vi "Save Settings.vi"(6 "Enable":bool, 8 "error in":errorcluster, 10 "Cluster":T1, 11 "VISA Refnum in":refnum<visa-resource-name>) -> (0 "error out":errorcluster, 2 "Cluster Out":T1, 3 "VISA out":refnum<visa-resource-name>)   [LabVIEW 2020]
uses:
  f6da1217-3e19-4b15-bc5f-b1b6cffed974.vi
  WriteSingleCoil.vi
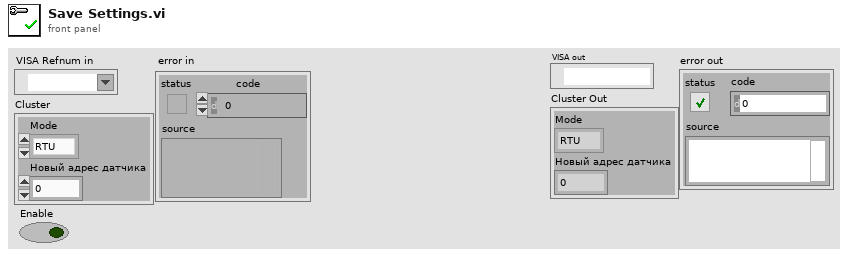
[diagram p1: front panel]
types:
  T1 = cluster{"Mode":enum16{"RTU", "ASCII"}, "Новый адрес датчика":u16}
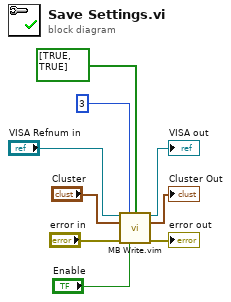
[diagram p0: block diagram]
diagram:
  n1 = call "MB Write.vim"("VISA Refnum in"="VISA Refnum in", "Command"=u16 3, "Data"=bool[] [TRUE, TRUE], "Cluster"="Cluster", "error in"="error in", "Enable"="Enable") -> ("VISA out"=→"VISA out":refnum<visa-resource-name>, "Cluster Out"=→"Cluster Out":T1, "error out"=→"error out":errorcluster)  [unwired: 7 in]
